vi "Deployment error handling.vi"(8 "error in (no error)":errorcluster) -> (0 "error out":errorcluster)   [LabVIEW 2013, in "PL Framework Configuration Tool.lvlib"]
uses:
  PL Framework Configuration Tool.lvlib
  <vilib>/Utility/error.llb/Error Cluster From Error Code.vi
  <vilib>/ErrorRing/Error Ring.xnode
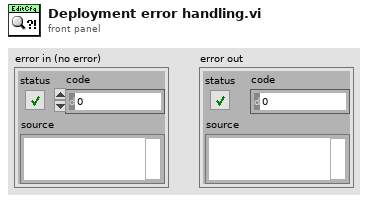
[diagram p1: front panel]
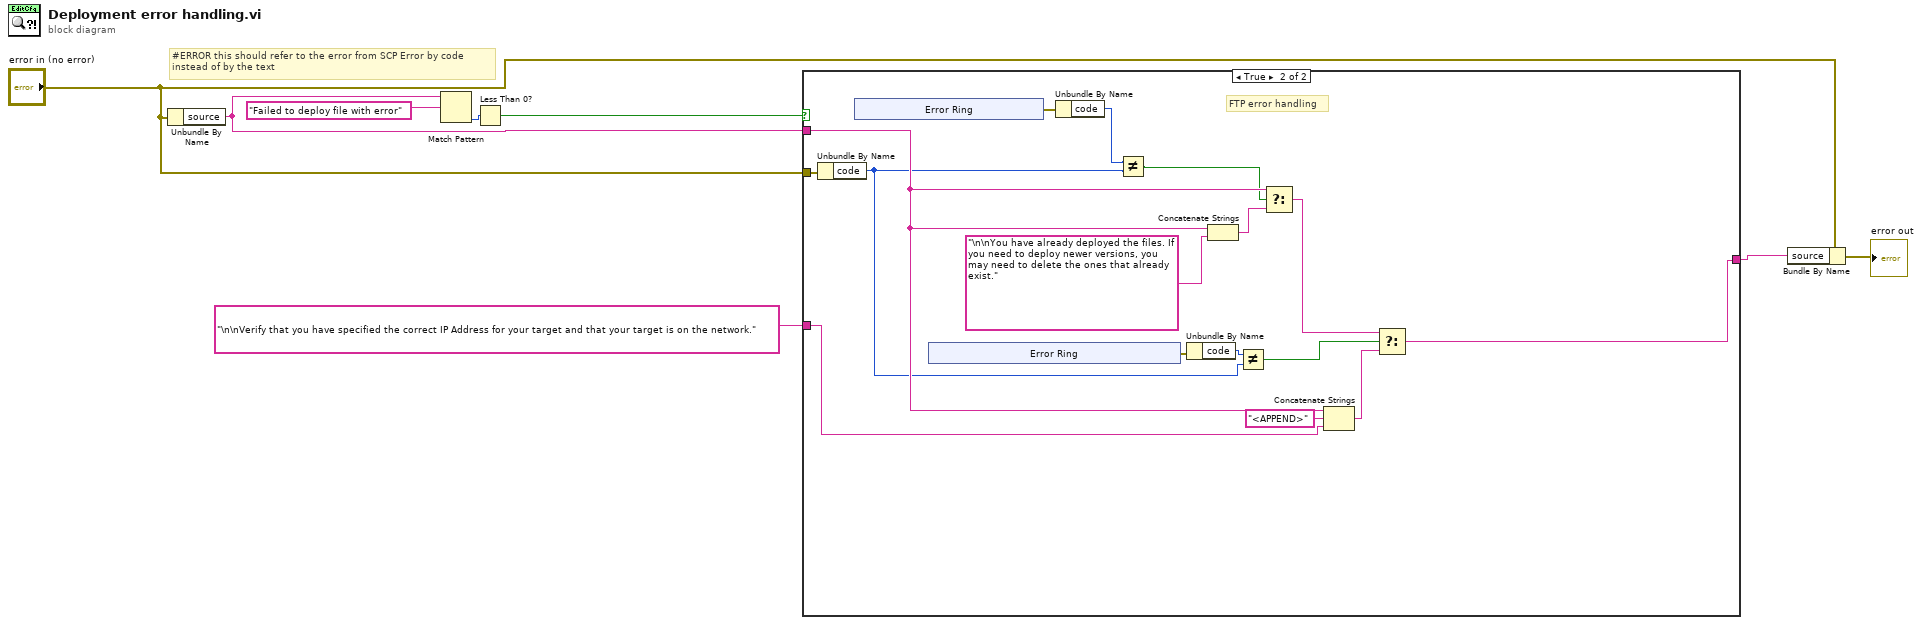
[diagram p0: block diagram]
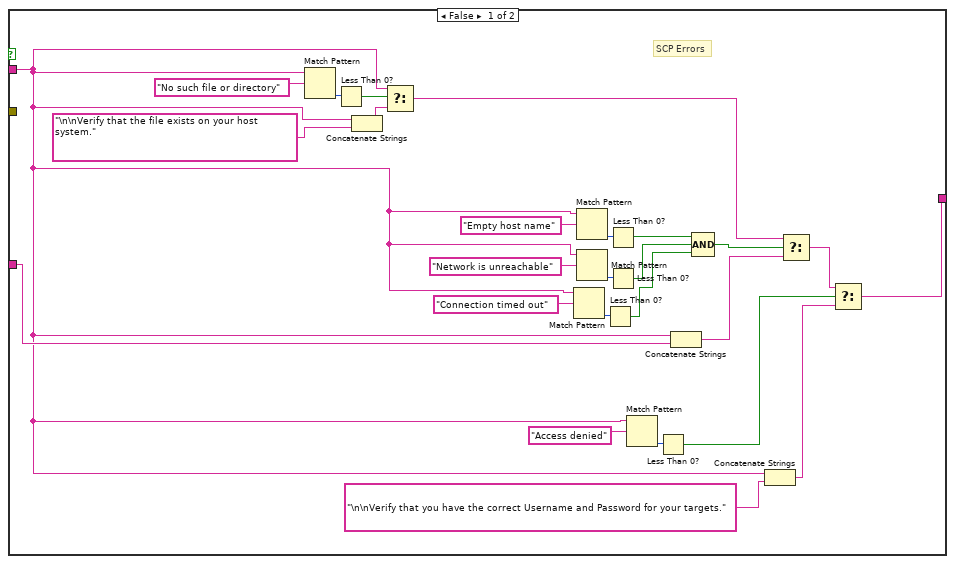
[diagram p2: hidden frame]
diagram:
  # "#ERROR this should refer to the error from SCP Error by code\ninstead of by the text"
  n1 = Unbundle By Name("error in (no error)") -> ("source"=w8:string)
  n2 = Match Pattern(string=w8, regular expression="Failed to deploy file with error") -> (offset past match=w6:i32)  [unwired: 1 in, 3 out]
  n3 = Less Than 0?(x=w6) -> (x < 0?=w7:bool)
  n4 = case shown="True" w7 {
    tunnel: w8 -> [w10 w47]
    tunnel: [w17 w44] -> w3
    tunnel: "\n\nVerify that you have specified the correct IP Address for your target and that your target is on the network." ("regular expression") -> [w16 w46]
    tunnel: "error in (no error)" -> [_ w40]
    frame False {
      # "SCP Errors"
      n5 = Match Pattern(string=w10, regular expression="No such file or directory") -> (offset past match=w15:i32)  [unwired: 1 in, 3 out]
      n6 = Less Than 0?(x=w15) -> (x < 0?=w13:bool)
      n7 = Concatenate Strings(w10, "\n\nVerify that the file exists on your host system." ("f")) -> (w9:string)
      n8 = Select(t=w10, s=w13, f=w9) -> (s? t:f=w12:string)
      n9 = Match Pattern(string=w10, regular expression="Connection timed out") -> (offset past match=w27:i32)  [unwired: 1 in, 3 out]
      n10 = Match Pattern(string=w10, regular expression="Empty host name") -> (offset past match=w33:i32)  [unwired: 1 in, 3 out]
      n11 = Match Pattern(string=w10, regular expression="Network is unreachable") -> (offset past match=w31:i32)  [unwired: 1 in, 3 out]
      n12 = Less Than 0?(x=w27) -> (x < 0?=w26:bool)
      n13 = Less Than 0?(x=w33) -> (x < 0?=w30:bool)
      n14 = Less Than 0?(x=w31) -> (x < 0?=w29:bool)
      n15 = Match Pattern(string=w10, regular expression="Access denied") -> (offset past match=w25:i32)  [unwired: 1 in, 3 out]
      n16 = Less Than 0?(x=w25) -> (x < 0?=w21:bool)
      n17 = Concatenate Strings(w10, w16) -> (w22:string)
      n18 = Compound Arithmetic op=AND(w30, w29, w26) -> (w23:bool)
      n19 = Concatenate Strings(w10, "\n\nVerify that you have the correct Username and Password for your targets." ("regular expression")) -> (w18:string)
      n20 = Select(t=w12, s=w23, f=w22) -> (s? t:f=w20:string)
      n21 = Select(t=w20, s=w21, f=w18) -> (s? t:f=w17:string)
    }
    frame True {
      # "FTP error handling"
      n22 = Unbundle By Name(w40) -> ("code"=w37:i32)
      n23 = xnode "Error Ring"() -> ("error out"=w41:errorcluster)
      n24 = xnode "Error Ring"() -> ("error out"=w39:errorcluster)
      n25 = Unbundle By Name(w41) -> ("code"=w42:i32)
      n26 = Not Equal?(x=w42, y=w37) -> (x != y?=w43:bool)
      n27 = Unbundle By Name(w39) -> ("code"=w38:i32)
      n28 = Concatenate Strings(w47, "\n\nYou have already deployed the files. If you need to deploy newer versions, you may need to delete the ones that already exist." ("regular expression")) -> (w49:string)
      n29 = Not Equal?(x=w38, y=w37) -> (x != y?=w36:bool)
      n30 = Select(t=w47, s=w43, f=w49) -> (s? t:f=w45:string)
      n31 = Concatenate Strings(w47, "<APPEND>" ("string"), w46) -> (w48:string)
      n32 = Select(t=w45, s=w36, f=w48) -> (s? t:f=w44:string)
    }
  }
  n33 = Bundle By Name(cluster="error in (no error)", "source"=w3) -> (→"error out":errorcluster)
